vi "Create_upload_and_erase_jlink.vi"(0 ".mot file":path, 1 "Password":string, 7 "path":path, 11 "error in":errorcluster) -> (15 "error out":errorcluster)   [LabVIEW 2023]
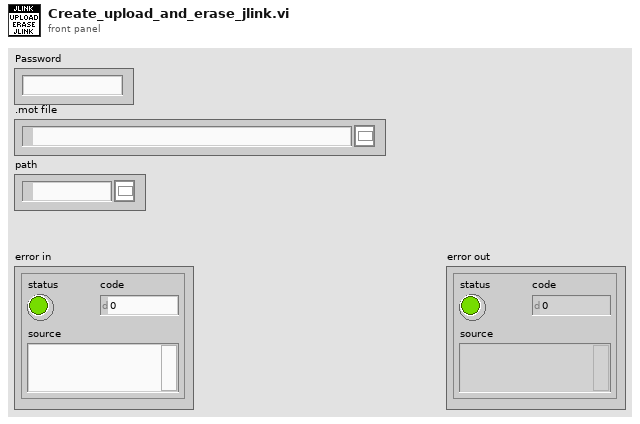
[diagram p1: front panel]
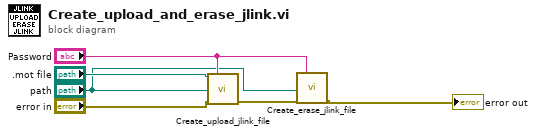
[diagram p0: block diagram]
diagram:
  n1 = call "Create_upload_jlink_file.vi"(".mot file"=".mot file", "Password"="Password", "path"="path", "error in"="error in") -> ("error out"=w6:errorcluster)  [unwired: 11 in]
  n2 = call "Create_erase_jlink_file.vi"("Password"="Password", "path"="path", "error in"=w6) -> ("error out"=→"error out":errorcluster)  [unwired: 12 in]
